vi "FM Set Amplitude.vi"(0 "Amplitude (V)":dbl format="%.1f") -> ()   [LabVIEW 2009]
uses:
  MWC Global.vi
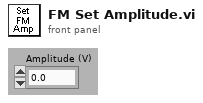
[diagram p1: front panel]
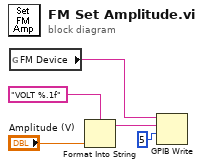
[diagram p0: block diagram]
diagram:
  n1 = global read "MWC Global.vi" "FM Device"() -> (w5:string)
  n2 = Format Into String(format string="VOLT %.1f" ("Format String"), "Amplitude (V)") -> (resulting string=w2:string)  [unwired: 2 in, 1 out]
  n3 = GPIB Write(0:w5, 1:w2, 2:i16 5 ("mode (0)")) -> ()  [unwired: 2 in, 2 out]
